vi "mainBeadAlignment.vi"() -> ()   [LabVIEW 2017]
uses:
  globalUtilities.vi
  globalDevices.vi
panel:
  in  "saveFrames":bool
  out "folder name":string
  out "frame":u16[][](graph)
  in  "stop":bool
  # "BEAD ALIGNMENT"
  # "Use xbox controller. If the recording\ndoes not start, click on this button <--"
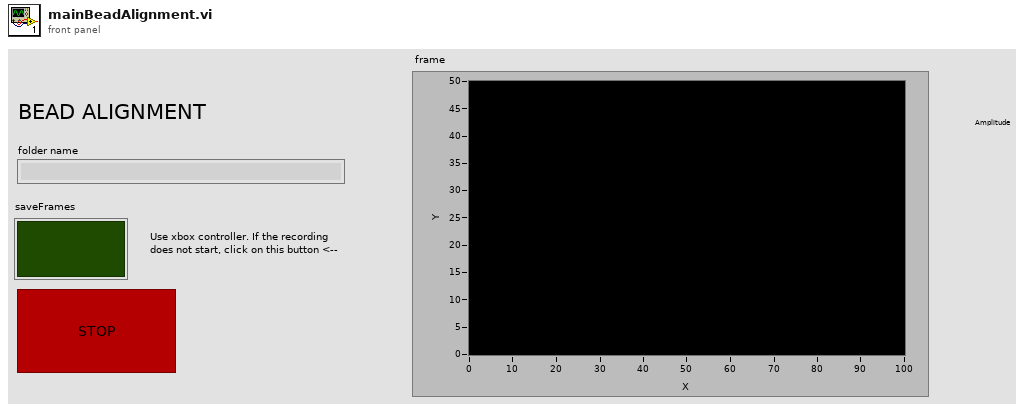
[diagram p1: front panel]
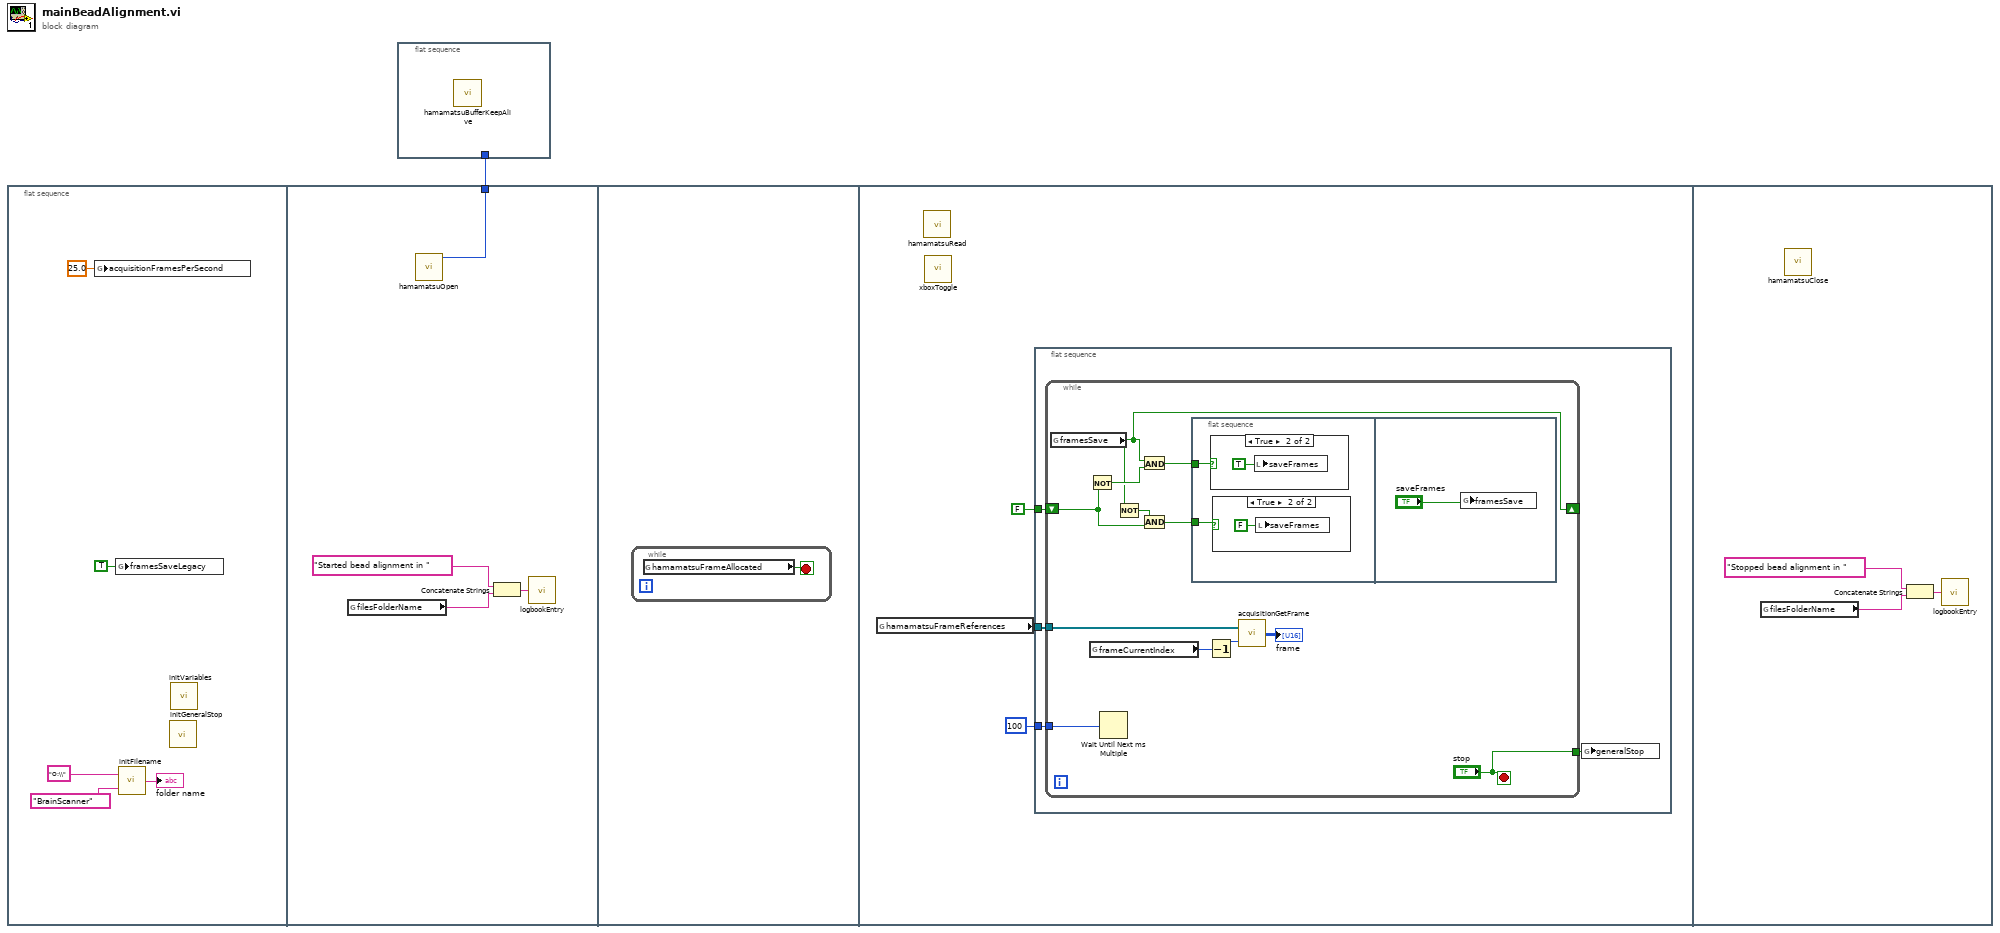
[diagram p0: block diagram]
diagram:
  n1 = flat-sequence {
    tunnel: [w7] -> w1
    frame #0 {
      n2 = global write "globalUtilities.vi" "acquisitionFramesPerSecond"(25.0 ("acquisitionFramesPerSecond")) -> ()
      n3 = global write "globalUtilities.vi" "framesSaveLegacy"(TRUE ("framesSaveLegacy")) -> ()
      n4 = call "initFilename.vi"("Experiment type"="BrainScanner", "Base disk and folder"="O:\\") -> ("folder name"=→"folder name":string)
      n5 = call "initGeneralStop.vi"() -> ()  [unwired: 1 in]
      n6 = call "initVariables.vi"() -> ()  [unwired: 12 in]
    }
    frame #1 {
      n7 = global read "globalUtilities.vi" "filesFolderName"() -> (w9:string)
      n8 = call "hamamatsuOpen.vi"() -> ("Handle out"=w7:u32)  [unwired: 3 out]
      n9 = Concatenate Strings("Started bead alignment in ", w9) -> (w10:string)
      n10 = call "logbookEntry.vi"("Log book entry"=w10) -> ()  [unwired: 2 out]
    }
    frame #2 {
      n11 = while {
        stop <- w11 stop-if-true
        n12 = global read "globalDevices.vi" "hamamatsuFrameAllocated"() -> (w11:bool)
      }
    }
    frame #3 {
      n13 = global read "globalDevices.vi" "hamamatsuFrameReferences"() -> (w14:refnum<data-value>[])
      n14 = call "hamamatsuRead.vi"() -> ()  [unwired: 12 in]
      n15 = call "xboxToggle.vi"() -> ()  [unwired: 12 in]
      n16 = flat-sequence {
        tunnel: w14 -> [w18]
        tunnel: u32 100 -> [w17]
        tunnel: FALSE -> [w15]
        frame #0 {
          n17 = while {
            tunnel: w18 -> [w30]
            tunnel: w17 -> [w28]
            tunnel: ["stop"] -> w16
            shift-right: [w19] -> _
            shift-left: w15 -> [w20]
            stop <- "stop" stop-if-true
            n18 = global read "globalUtilities.vi" "framesSave"() -> (w19:bool)
            n19 = Not(x=w20) -> (.not. x?=w24:bool)
            n20 = global read "globalUtilities.vi" "frameCurrentIndex"() -> (w26:i32)
            n21 = Wait Until Next ms Multiple(millisecond multiple=w28) -> ()  [unwired: 1 out]
            n22 = Not(x=w19) -> (.not. x?=w22:bool)
            n23 = And(x=w19, y=w24) -> (x .and. y?=w23:bool)
            n24 = And(x=w22, y=w20) -> (x .and. y?=w21:bool)
            n25 = flat-sequence {
              tunnel: w23 -> [w32]
              tunnel: w21 -> [w31]
              frame #0 {
                n26 = case shown="True" w32 {
                  frame False {
                  }
                  frame True {
                    n27 = local write "saveFrames"(TRUE ("saveFrames")) -> ()
                  }
                }
                n28 = case shown="True" w31 {
                  frame False {
                  }
                  frame True {
                    n29 = local write "saveFrames"(FALSE ("saveFrames")) -> ()
                  }
                }
              }
              frame #1 {
                n30 = global write "globalUtilities.vi" "framesSave"("saveFrames") -> ()
              }
            }
            n31 = Decrement(x=w26) -> (x-1=w25:i32)
            n32 = call "acquisitionGetFrame.vi"("index"=w25, "hamamatsuFrameReferences"=w30) -> ("frameOut"=→"frame":u16[][])
          }
          n33 = global write "globalUtilities.vi" "generalStop"(w16) -> ()
        }
      }
    }
    frame #4 {
      n34 = global read "globalUtilities.vi" "filesFolderName"() -> (w37:string)
      n35 = call "hamamatsuClose.vi"() -> ()  [unwired: 1 out]
      n36 = Concatenate Strings("Stopped bead alignment in ", w37) -> (w36:string)
      n37 = call "logbookEntry.vi"("Log book entry"=w36) -> ()  [unwired: 2 out]
    }
  }
  n38 = flat-sequence {
    tunnel: w1 -> [_]
    frame #0 {
      n39 = call "hamamatsuBufferKeepAlive.vi"() -> ()  [unwired: 12 in]
    }
  }
